vi "test_libssh2_sftp_readdir.vi"() -> ()   [LabVIEW 2013, in "libssh2_integration_tests.lvlib"]
uses:
  libssh2_integration_tests.lvlib
  <vilib>/addons/_JKI Toolkits/Caraya/classes/Test/Test.lvclass
  support/support.lvlib
  libssh2/libssh2.lvlib
  <vilib>/addons/_JKI Toolkits/Caraya/classes/Assert/Assert.lvclass
panel:
  out "error out":errorcluster
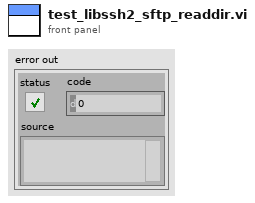
[diagram p1: front panel]
types:
  T1 = typedef "libssh2.lvlib/Session Refnum.ctl" = refnum<k1>
  T2 = typedef "libssh2.lvlib/SFTP Refnum.ctl" = refnum<k1>
  T3 = typedef "libssh2.lvlib/SFTP Handle Refnum.ctl" = refnum<k1>
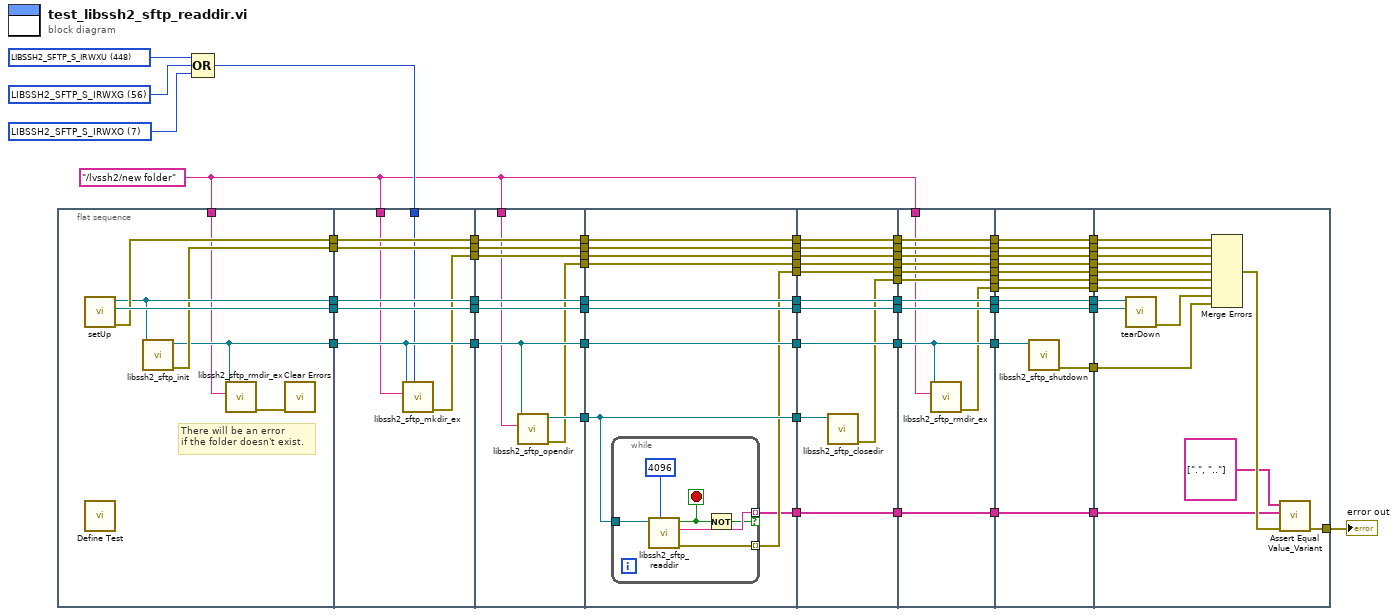
[diagram p0: block diagram]
diagram:
  w3 = "/lvssh2/new folder" ("filename")
  w59 = 7 items=["LIBSSH2_SFTP_S_IRWXU"=448, "LIBSSH2_SFTP_S_IRUSR"=256, "LIBSSH2_SFTP_S_IWUSR"=128, "LIBSSH2_SFTP_S_IXUSR"=64, "LIBSSH2_SFTP_S_IRWXG"=56, "LIBSSH2_SFTP_S_IRGRP"=32, "LIBSSH2_SFTP_S_IWGRP"=16, "LIBSSH2_SFTP_S_IXGRP"=8, "LIBSSH2_SFTP_S_IRWXO"=7, "LIBSSH2_SFTP_S_IROTH"=4, "LIBSSH2_SFTP_S_IWOTH"=2, "LIBSSH2_SFTP_S_IXOTH"=1] ("mode")
  w60 = 56 items=["LIBSSH2_SFTP_S_IRWXU"=448, "LIBSSH2_SFTP_S_IRUSR"=256, "LIBSSH2_SFTP_S_IWUSR"=128, "LIBSSH2_SFTP_S_IXUSR"=64, "LIBSSH2_SFTP_S_IRWXG"=56, "LIBSSH2_SFTP_S_IRGRP"=32, "LIBSSH2_SFTP_S_IWGRP"=16, "LIBSSH2_SFTP_S_IXGRP"=8, "LIBSSH2_SFTP_S_IRWXO"=7, "LIBSSH2_SFTP_S_IROTH"=4, "LIBSSH2_SFTP_S_IWOTH"=2, "LIBSSH2_SFTP_S_IXOTH"=1] ("mode")
  w61 = 448 items=["LIBSSH2_SFTP_S_IRWXU"=448, "LIBSSH2_SFTP_S_IRUSR"=256, "LIBSSH2_SFTP_S_IWUSR"=128, "LIBSSH2_SFTP_S_IXUSR"=64, "LIBSSH2_SFTP_S_IRWXG"=56, "LIBSSH2_SFTP_S_IRGRP"=32, "LIBSSH2_SFTP_S_IWGRP"=16, "LIBSSH2_SFTP_S_IXGRP"=8, "LIBSSH2_SFTP_S_IRWXO"=7, "LIBSSH2_SFTP_S_IROTH"=4, "LIBSSH2_SFTP_S_IWOTH"=2, "LIBSSH2_SFTP_S_IXOTH"=1] ("mode")
  n1 = flat-sequence {
    tunnel: [w72] -> w67
    tunnel: [w74] -> w66
    tunnel: [w73] -> w65
    tunnel: [w71] -> w63
    tunnel: [w70] -> w62
    tunnel: w3 -> [w69]
    tunnel: w67 -> [w82]
    tunnel: w66 -> [w81]
    tunnel: [w82] -> w50
    tunnel: [w81] -> w49
    tunnel: [w78] -> w48
    tunnel: [w80] -> w47
    tunnel: w65 -> [w80]
    tunnel: w63 -> [w79]
    tunnel: [w79] -> w46
    tunnel: w62 -> [w78]
    tunnel: w58 -> [w77]
    tunnel: w3 -> [w76]
    tunnel: [w75] -> w45
    tunnel: w50 -> [w91]
    tunnel: [w91] -> w42
    tunnel: w49 -> [w90]
    tunnel: [w90] -> w40
    tunnel: w48 -> [w86]
    tunnel: [w86] -> w38
    tunnel: w47 -> [w89]
    tunnel: [w89] -> w36
    tunnel: w46 -> [w88]
    tunnel: [w88] -> w34
    tunnel: w45 -> [w87]
    tunnel: [w87] -> w32
    tunnel: w3 -> [w85]
    tunnel: [w84] -> w30
    tunnel: [w83] -> w28
    tunnel: w42 -> [w101]
    tunnel: [w101] -> w41
    tunnel: w40 -> [w100]
    tunnel: [w100] -> w39
    tunnel: w38 -> [w99]
    tunnel: [w99] -> w37
    tunnel: w36 -> [w98]
    tunnel: [w98] -> w35
    tunnel: w34 -> [w97]
    tunnel: [w97] -> w33
    tunnel: w32 -> [w96]
    tunnel: [w96] -> w31
    tunnel: w30 -> [w94]
    tunnel: [w94] -> w29
    tunnel: w28 -> [w95]
    tunnel: [w95] -> w27
    tunnel: [w93] -> w26
    tunnel: [w92] -> w24
    tunnel: w41 -> [w118]
    tunnel: [w118] -> w23
    tunnel: w39 -> [w117]
    tunnel: [w117] -> w21
    tunnel: w37 -> [w116]
    tunnel: [w116] -> w19
    tunnel: w35 -> [w115]
    tunnel: [w115] -> w17
    tunnel: w33 -> [w114]
    tunnel: [w114] -> w15
    tunnel: w31 -> [w113]
    tunnel: [w113] -> w13
    tunnel: w29 -> [w112]
    tunnel: [w108] -> w11
    tunnel: w27 -> [w111]
    tunnel: [w111] -> w9
    tunnel: [w110] -> w7
    tunnel: w26 -> [w109]
    tunnel: [w109] -> w5
    tunnel: w24 -> [w108]
    tunnel: w23 -> [w130]
    tunnel: [w130] -> w22
    tunnel: w21 -> [w129]
    tunnel: [w129] -> w20
    tunnel: w19 -> [w121]
    tunnel: [w121] -> w18
    tunnel: w17 -> [w128]
    tunnel: [w128] -> w16
    tunnel: w15 -> [w127]
    tunnel: [w127] -> w14
    tunnel: w13 -> [w126]
    tunnel: [w126] -> w12
    tunnel: w11 -> [w125]
    tunnel: [w125] -> w10
    tunnel: w9 -> [w124]
    tunnel: [w124] -> w8
    tunnel: w7 -> [w123]
    tunnel: [w123] -> w6
    tunnel: w5 -> [w122]
    tunnel: [w122] -> w4
    tunnel: w3 -> [w120]
    tunnel: [w119] -> w2
    tunnel: w22 -> [w142]
    tunnel: [w142] -> w57
    tunnel: w20 -> [w141]
    tunnel: [w141] -> w56
    tunnel: w18 -> [w138]
    tunnel: [w135] -> w55
    tunnel: w16 -> [w140]
    tunnel: [w140] -> w54
    tunnel: w14 -> [w139]
    tunnel: [w139] -> w53
    tunnel: [w137] -> w52
    tunnel: w12 -> [w136]
    tunnel: [w136] -> w51
    tunnel: [w134] -> w44
    tunnel: w10 -> [w135]
    tunnel: w8 -> [w134]
    tunnel: w6 -> [w133]
    tunnel: [w133] -> w43
    tunnel: w4 -> [w132]
    tunnel: [w132] -> w25
    tunnel: w2 -> [w131]
    tunnel: [w131] -> w1
    tunnel: w57 -> [w157]
    tunnel: w56 -> [w156]
    tunnel: w55 -> [w145]
    tunnel: w54 -> [w155]
    tunnel: [w152] -> w64
    tunnel: w53 -> [w151]
    tunnel: w52 -> [w150]
    tunnel: w51 -> [w149]
    tunnel: w44 -> [w148]
    tunnel: w43 -> [w147]
    tunnel: w25 -> [w146]
    tunnel: w1 -> [w143]
    frame #0 {
      # "There will be an error\nif the folder doesn't exist."
      n2 = call "setUp.vi"() -> ("error out"=w73:errorcluster, "connection ID"=w74:refnum<k5>, "session"=w72:T1)  [unwired: 9 in]
      n3 = call <vilib>:"Define Test.vi"() -> ()  [unwired: 10 in, 2 out]
      n4 = call "libssh2_sftp_init.vi"("session"=w72) -> ("error out"=w71:errorcluster, "sftp"=w70:T2)  [unwired: 9 in]
      n5 = call "libssh2_sftp_rmdir_ex.vi"("path"=w69, "sftp"=w70) -> ("error out"=w68:errorcluster)  [unwired: 9 in]
      n6 = call <vilib>:"Clear Errors.vi"("error in (no error)"=w68) -> ()  [unwired: 6 in, 1 out]
    }
    frame #1 {
      n7 = call "libssh2_sftp_mkdir_ex.vi"("mode"=w77, "path"=w76, "sftp"=w78) -> ("error out"=w75:errorcluster)  [unwired: 8 in]
    }
    frame #2 {
      n8 = call "libssh2_sftp_opendir.vi"("path"=w85, "sftp"=w86) -> ("error out"=w83:errorcluster, "sftp handle"=w84:T3)  [unwired: 8 in]
    }
    frame #3 {
      n9 = while {
        tunnel: w94 -> [w107]
        tunnel: [w105] -> w93 mode=indexing
        tunnel: [w104] -> w92 mode=indexing if=w102
        stop <- w103 stop-if-true
        n10 = call "libssh2_sftp_readdir.vi"("buffer maxlen"=4096, "sftp handle"=w107) -> ("error out"=w105:errorcluster, "buffer"=w104:string, "no more files"=w103:bool)  [unwired: 6 in, 1 out]
        n11 = Not(x=w103) -> (.not. x?=w102:bool)
      }
    }
    frame #4 {
      n12 = call "libssh2_sftp_closedir.vi"("sftp handle"=w112) -> ("error out"=w110:errorcluster)  [unwired: 10 in]
    }
    frame #5 {
      n13 = call "libssh2_sftp_rmdir_ex.vi"("path"=w120, "sftp"=w121) -> ("error out"=w119:errorcluster)  [unwired: 9 in]
    }
    frame #6 {
      n14 = call "libssh2_sftp_shutdown.vi"("sftp"=w138) -> ("error out"=w137:errorcluster)  [unwired: 10 in]
    }
    frame #7 {
      n15 = call "tearDown.vi"("connection ID"=w156, "session"=w157) -> ("error out"=w154:errorcluster)  [unwired: 9 in]
      n16 = Merge Errors(w155, w151, w149, w148, w146, w147, w143, w154, w150) -> (w153:errorcluster)
      n17 = call <vilib>:"Assert Equal Value_Variant.vi"("error in (no error)"=w153, "Y"=w145, "X"=string[] [".", ".."]) -> ("error out"=w152:errorcluster)  [unwired: 7 in, 1 out]
    }
  }
  n18 = Compound Arithmetic op=OR(w61, w60, w59) -> (w58:i32)
  "error out" <- w64
